vi "Expt8b_MT Block Interleaver-DeInterleaver_Student_lab.vi"() -> ()   [LabVIEW 2020]
doc: "This example demonstrates the programming of block Interleaver and Deinterleaver. \nNOTE : The number of elements in \"Interleaved Symbols\" and \"Deinterleaved Symbols\" arrays will be N=(number of rows)*(number of columns)*int[(Number of Message Symbols)/(number of rows*number of columns)]. \nFor example if, \nNumber of Message Symbols = 1000 \nNumber of Rows = 3\nNumber of Columns = 4 \nN=int[1000/(3*4)]=12*int[1000/12]=996"
uses:
  <vilib>/addons/Modulation/Digital/General/MT Generate Bits (Galois, PN Order).vi
  <vilib>/addons/Modulation/Digital/Support/Common/Validators/mod_Generate Bits Validate.vi
  <vilib>/addons/Modulation/Analog/support/mod_Set Error Source.vi
  <vilib>/addons/Modulation/Digital/General/subVIs/mod_Generate Bits PN Sequence.vi
  <vilib>/addons/Modulation/niDMT.lvlib
panel:
  in  "Number of Columns":i32=3
  in  "Number of Rows":i32=2
  out "Deinterleaved Symbols":i32[](array[numeric])
  out "Error Out":errorcluster
  out "Message Symbols":i32[](array[numeric])
  out "Interleaved Symbols":i32[](array[numeric])
  in  "Number of Message Symbols":i32=1000
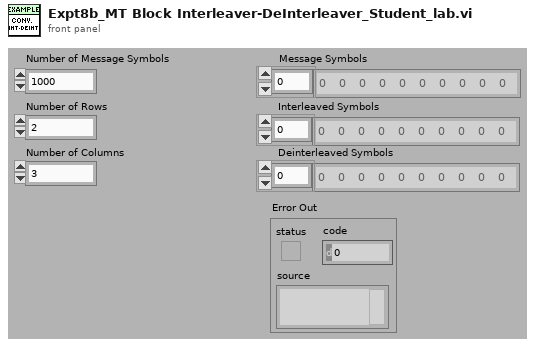
[diagram p1: front panel]
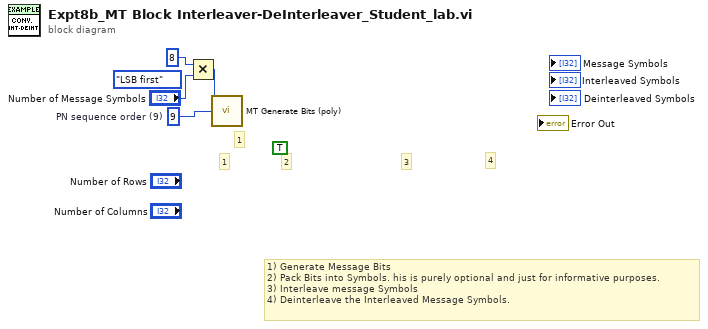
[diagram p0: block diagram]
diagram:
  (unwired) TRUE ("reset ? (T)")
  (unwired) enum16{"MSB first", "LSB first"}."LSB first" ("packed bit order")
  w4 = 9  # PN sequence order (9)
  # "4"
  # "3"
  # "2"
  # "1"
  # "1"
  # "1) Generate Message Bits\n2) Pack Bits into Symbols. his is purely optional and just for informative purposes. \n3) Interleave message Symbols\n4) Deinterleave the Interleaved Message Symbols."
  n1 = Multiply(x=8 ("bits per integer"), y="Number of Message Symbols") -> (x*y=w1:i32)
  n2 = call-poly <vilib>:"MT Generate Bits (poly).vi"("total bits (128)"=w1, "PN sequence order (9)"=w4) -> ()  [unwired: 11 in, 3 out]
